vi "Open Pane.vi"(7 "vi refnum":refnum<vi>, 8 "error in":errorcluster {"code" format="%.0x"}) -> (0 "error out":errorcluster {"code" format="%.0x"}, 3 "connect pane":refnum<vi>, 5 "vi refnum out":refnum<vi>)   [LabVIEW 2018, in "NISAST VI Scripting.lvlib" / "VI.lvlib" / "Connector.lvlib"]
uses:
  Connector.lvlib
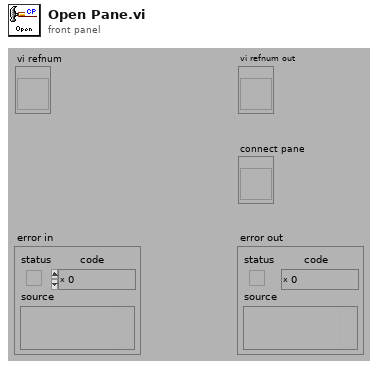
[diagram p1: front panel]
types:
  T1 = typedef "NISAST VI Scripting.lvlib/VI.lvlib/Front Panel.lvlib/Connector Pane Type.ctl" = enum16{"4-2-2-4", "5-2-2-2-5", "Others"}
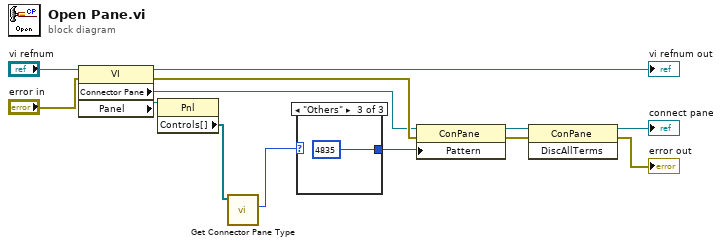
[diagram p0: block diagram]
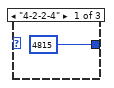
[diagram p2: hidden frame]
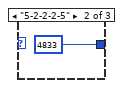
[diagram p3: hidden frame]
diagram:
  n1 = property class="VI"(reference="vi refnum", error in="error in") -> (reference out=→"vi refnum out":refnum<vi>, error out=w8:errorcluster, "Connector Pane"=w7:refnum<vi>, "Panel"=w4:refnum<vi>)
  n2 = property class="Pnl"(reference=w4) -> ("Controls[]"=w2:refnum<vi>[])  [unwired: 1 in, 2 out]
  n3 = call "Get Connector Pane Type.vi"("Controls[]"=w2) -> ("Connector Pane Type"=w1:T1)  [unwired: 1 in, 8 out]
  n4 = case shown="\"Others\"" w1 {
    tunnel: [u32 4815 ("Pattern") u32 4833 ("Pattern") u32 4835 ("Pattern")] -> w3
    frame "4-2-2-4" {
    }
    frame "5-2-2-2-5" {
    }
    frame "Others" {
    }
  }
  n5 = property class="ConPane"(reference=w7, error in=w8, "Pattern"=w3) -> (reference out=w10:refnum<vi>, error out=w9:errorcluster)
  n6 = invoke class="ConPane" method="DiscAllTerms"(reference=w10, error in=w9) -> (reference out=→"connect pane":refnum<vi>, error out=→"error out":errorcluster)  [unwired: 1 in, 1 out]
